vi "GetBeamDiameter.vi"(3 "resource name":string="USB0::0x1313::0x8078::P0005368::INSTR") -> (0 "error out":errorcluster {"code" format="%.0x"}, 1 "Beam Diameter (sq mm):":dbl caption="Beam Diameter")   [LabVIEW 2015]
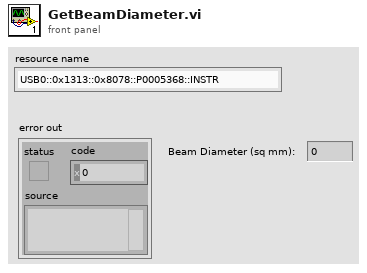
[diagram p1: front panel]
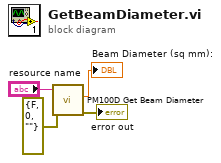
[diagram p0: block diagram]
diagram:
  n1 = call "PM100D Get Beam Diameter.vi"("error in (no error)"=errorcluster {"status"=FALSE, "code"=0, "source"=""}, "instrument handle"="resource name") -> ("error out"=→"error out":errorcluster, "Beam Diameter"=→"Beam Diameter (sq mm):":dbl)  [unwired: 7 in, 1 out]
